vi "tkrsa6100 Binary to 32 int.vi"(11 "Substring":string) -> (3 "String":string)   [LabVIEW 2020, in "Library Instrument & Equipement.lvlib" / "Library Spectrum Analyser.lvlib"]
uses:
  Library Spectrum Analyser.lvlib
panel:
  # "RSA6100 Binary to 32 Bit Int  Converter"
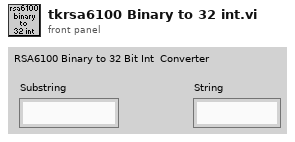
[diagram p1: front panel]
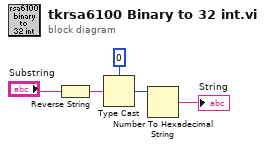
[diagram p0: block diagram]
diagram:
  n1 = Reverse String(1:"Substring") -> (0:w4:string)
  n2 = Type Cast(type=u32 0 ("default (0 I32)"), x=w4) -> (*(type *) &x=w2:u32)
  n3 = Number To Hexadecimal String(2:w2) -> (0:→"String":string)  [unwired: 1 out]
